vi "Define Home Motor.vi"(6 "Home Position (0 units)":dbl min=-2000000000.0 max=2000000000.0 format="%.4g", 8 "error in (no error)":errorcluster, 9 "Axis (1)":i32=1 min=1 max=3, 10 "VISA resource name":refnum<visa-resource-name>, 11 "ESP302 in":refnum<class "ESP302.lvclass">) -> (0 "error out":errorcluster, 2 "VISA resource name out":refnum<visa-resource-name>, 3 "ESP302 out":refnum<class "ESP302.lvclass">)   [LabVIEW 2020, in "ESP302.lvclass"]
uses:
  ESP302.lvclass
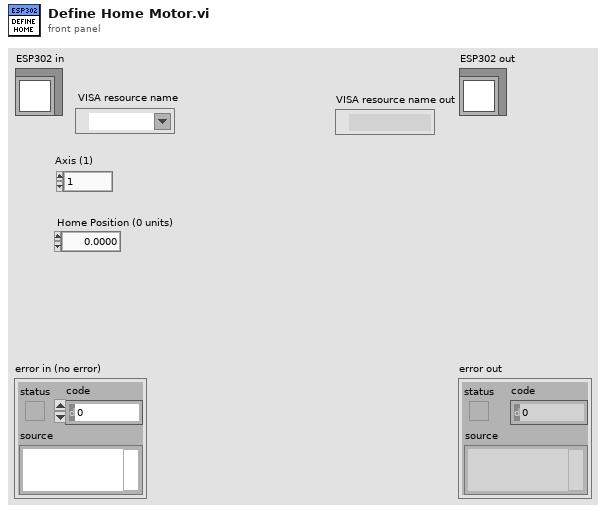
[diagram p1: front panel]
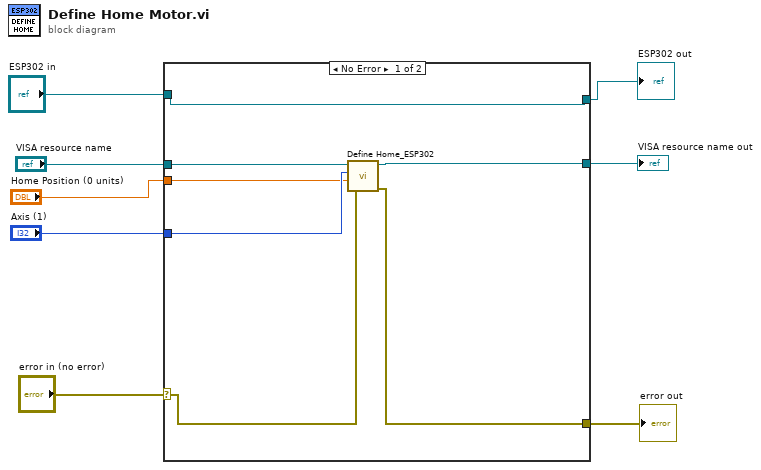
[diagram p0: block diagram]
diagram:
  n1 = case shown="No Error" "error in (no error)" {
    selector: "error in (no error)" -> [w11 w18]
    tunnel: [w10 w18] -> w7
    tunnel: "VISA resource name" -> [w15 w17]
    tunnel: [w14 w17] -> w5
    tunnel: "Axis (1)" -> [w13 _]
    tunnel: "Home Position (0 units)" -> [w12 _]
    tunnel: [w9 w16] -> w1
    tunnel: "ESP302 in" -> [w9 w16]
    frame No Error {
      n2 = call "Define Home_ESP302.vi"("error in (no error)"=w11, "Home Position (0 units)"=w12, "Axis (1)"=w13, "VISA resource name"=w15) -> ("error out"=w10:errorcluster, "VISA resource name out"=w14:refnum<visa-resource-name>)  [unwired: 2 in]
    }
    frame Error {
    }
  }
  "error out" <- w7
  "ESP302 out" <- w1
  "VISA resource name out" <- w5
